vi "Line Following.vi"(11 "Sensor Array":bool[](array[boolean])) -> (3 "Motor Values":dbl[](array[numeric]))   [LabVIEW 2018]
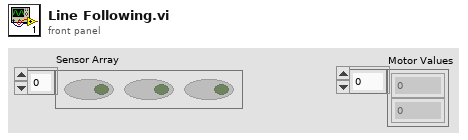
[diagram p1: front panel]
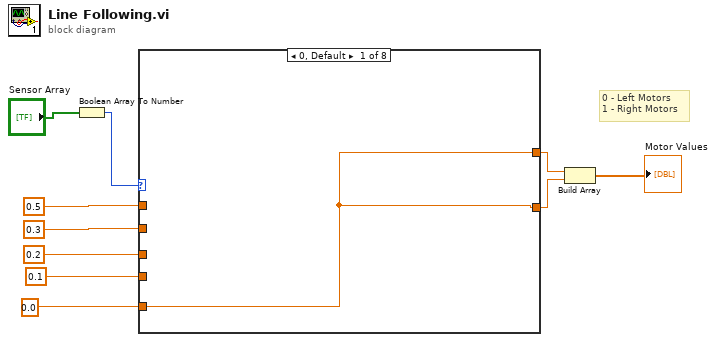
[diagram p0: block diagram]
diagram:
  # "0 - Left Motors\n1 - Right Motors"
  n1 = Boolean Array To Number(Boolean array="Sensor Array") -> (number=w9:u32)
  n2 = case shown="0, Default" w9 {
    tunnel: 0.0 -> [w11 _ _ _ _ w19 _ w22]
    tunnel: [w11 w13 w14 w15 w17 w19 w20 w22] -> w6
    tunnel: [w11 w12 w14 w16 w18 w19 w21 w22] -> w5
    tunnel: 0.1 -> [_ w12 _ w16 w17 _ w20 _]
    tunnel: 0.3 -> [_ w13 _ _ w18 _ _ _]
    tunnel: 0.5 -> [_ _ w14 _ _ _ _ _]
    tunnel: 0.2 -> [_ _ _ w15 _ _ w21 _]
    frame 0, Default {
    }
    frame 1 {
    }
    frame 2 {
    }
    frame 3 {
    }
    frame 4 {
    }
    frame 5 {
    }
    frame 6 {
    }
    frame 7 {
    }
  }
  n3 = Build Array(w6, w5) -> (→"Motor Values":dbl[])
